vi "Modbus Search For Message.vi"(4 "Test chamber is in sequence - LDO":bool, 6 "Test chamber is in sequence - FVIR":bool, 8 "error in (no error)":errorcluster, 10 "Message":string, 11 "Modbus Input":refnum<queue>) -> (0 "error out":errorcluster, 2 "Loop Rate":u32, 3 "Modbus Output":refnum<queue>)   [LabVIEW 2023, in "Modbus.lvlib"]
uses:
  Modbus.lvlib
  support/Message Queue/Message Cluster.ctl
  support/Message Queue/Enqueue Message (Single).vi
  support/Message Queue/Message Queue.lvlib
panel:
  out "elements":T1[](array[typedef])
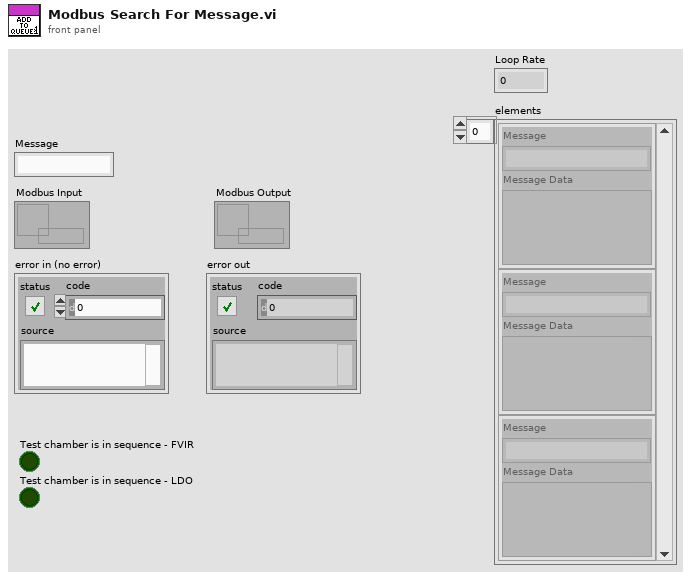
[diagram p1: front panel]
types:
  T1 = typedef "Message Queue.lvlib/Message Cluster.ctl" = cluster{"Message":string, "Message Data":variant}
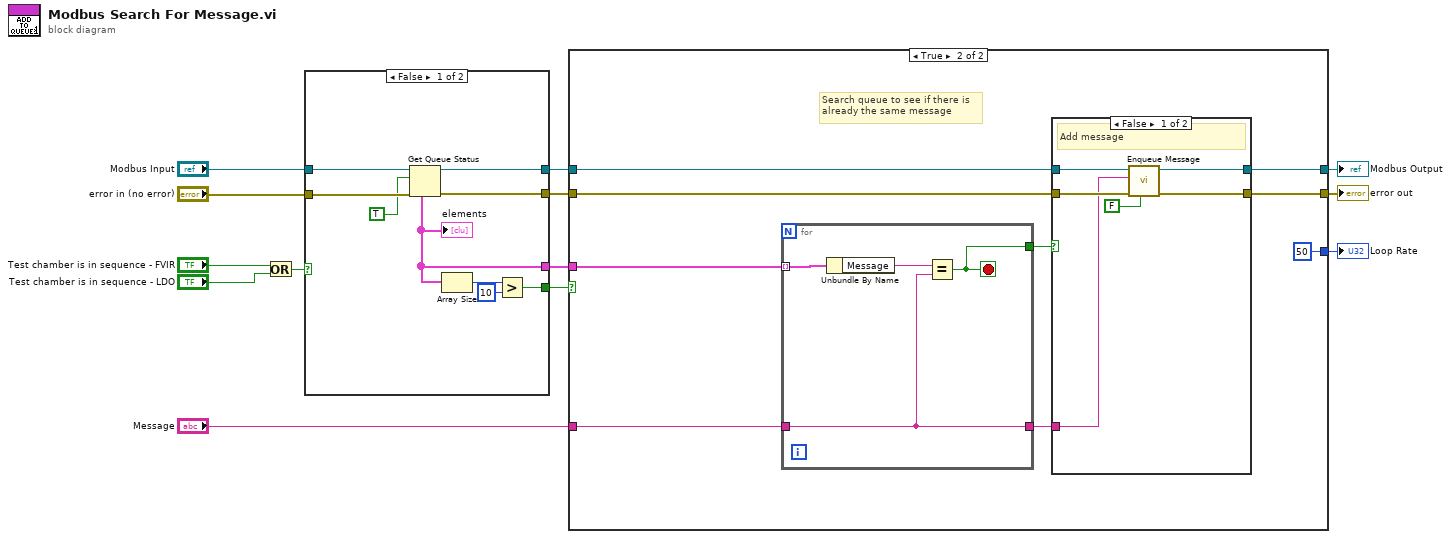
[diagram p0: block diagram]
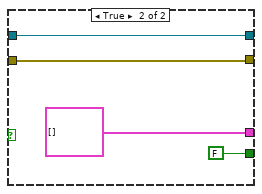
[diagram p2: hidden frame]
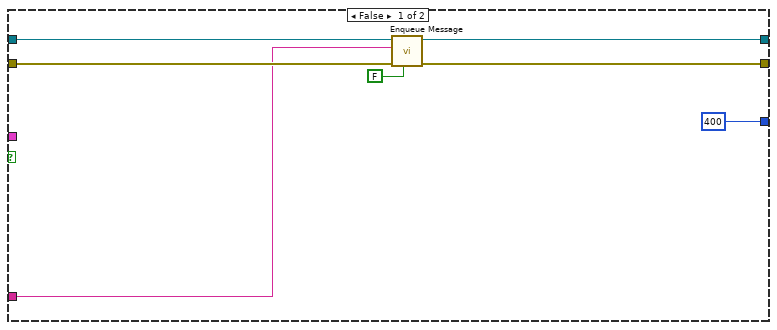
[diagram p3: hidden frame]
diagram:
  n1 = Or(x="Test chamber is in sequence - FVIR", y="Test chamber is in sequence - LDO") -> (x .or. y?=w1:bool)
  n2 = case shown="False" w1 {
    tunnel: "error in (no error)" -> [w22 w25]
    tunnel: "Modbus Input" -> [w20 w26]
    tunnel: [w19 w25] -> w11
    tunnel: [w18 w26] -> w10
    tunnel: [w17 T1[] [] ("elements")] -> w7
    tunnel: [w14 FALSE] -> w5
    frame False {
      n3 = Get Queue Status(queue=w20, return elements? (F)=TRUE, error in (no error)=w22) -> (queue out=w18:refnum<queue>, error out=w19:errorcluster, elements=w17:T1[])  [unwired: 5 out]
      "elements" <- w17
      n4 = Array Size(array=w17) -> (size(s)=w16:i32)
      n5 = Greater?(x=w16, y=10) -> (0:w14:bool)
    }
    frame True {
    }
  }
  n6 = case shown="True" w5 {
    tunnel: w7 -> [_ w42]
    tunnel: "Message" -> [w28 w41]
    tunnel: w11 -> [w30 w40]
    tunnel: w10 -> [w32 w38]
    tunnel: [w29 w37] -> w9
    tunnel: [w31 w36] -> w8
    tunnel: [u32 400 ("Read") u32 50 ("Read")] -> w4
    frame False {
      n7 = call-poly "Enqueue Message.vi"("Priority Message? (F)"=FALSE, "error in (no error)"=w30, "Message"=w28, "Message Queue"=w32) -> ("error out"=w29:errorcluster, "dup Message Queue"=w31:refnum<queue>)  [unwired: 6 in]
    }
    frame True {
      # "Search queue to see if there is \nalready the same message"
      n8 = for {
        tunnel: w42 -> [w54] mode=indexing
        tunnel: w41 -> [w51]
        tunnel: [w52] -> w39
        tunnel: [w51] -> w35
        stop <- w52 stop-if-true
        n9 = Unbundle By Name(w54) -> ("Message"=w53:string)
        n10 = Equal?(x=w53, y=w51) -> (x = y?=w52:bool)
      }
      n11 = case shown="False" w39 {
        tunnel: w40 -> [w47 w49]
        tunnel: w38 -> [w46 w50]
        tunnel: [w45 w50] -> w36
        tunnel: [w44 w49] -> w37
        tunnel: w35 -> [w43 _]
        frame False {
          # "Add message"
          n12 = call-poly "Enqueue Message.vi"("Priority Message? (F)"=FALSE, "error in (no error)"=w47, "Message"=w43, "Message Queue"=w46) -> ("error out"=w44:errorcluster, "dup Message Queue"=w45:refnum<queue>)  [unwired: 6 in]
        }
        frame True {
          # "If there is already a message, no need to add another."
        }
      }
    }
  }
  "error out" <- w9
  "Modbus Output" <- w8
  "Loop Rate" <- w4
